vi "Arm Solenoid.vi"(10 "Value":T1, 11 "Enum":enum16{"Start", "Run", "End"}(ring)=enum."Run") -> ()   [LabVIEW 2012]
uses:
  TypeDefs/Solenoid Module 1.ctl
  <vilib>/Rock Robotics/WPI/Solenoid/WPI_SolenoidChannel.ctl
  <vilib>/Rock Robotics/SystemInterfaces/Typedef/FPGA_TypedefSolenoidModule.ctl
  <vilib>/Rock Robotics/WPI/Solenoid/WPI_SolenoidValue.ctl
  <vilib>/Rock Robotics/WPI/Solenoid/WPI_SolenoidOpenDouble.vi
  <vilib>/Rock Robotics/WPI/Solenoid/WPI_SolenoidSetEnum.vi
panel:
  in  "Solenoid Module 1":T2={"Lock Arm"=enum."Solenoid 1", "Shoot FWD"=enum."Solenoid 2", "Shoot REV"=enum."Solenoid 3", "Tip FWD"=enum."Solenoid 4", "Tip REV"=enum."Solenoid 5", "Unassigned"=enum."Solenoid 6", "Unassigned"=enum."Solenoid 7", "Unassigned"=enum."Solenoid 8", "Module"=enum."Solenoid Module 1"}
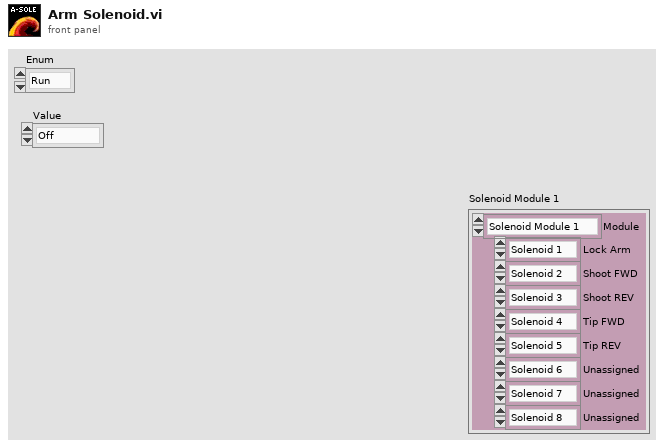
[diagram p1: front panel]
types:
  T1 = typedef "WPI_SolenoidValue.ctl" = enum16{"Off", "On", "Forward", "Reverse"}
  T2 = typedef "Solenoid Module 1.ctl" = cluster{"Lock Arm":T3, "Shoot FWD":T3, "Shoot REV":T3, "Tip FWD":T3, "Tip REV":T3, "Unassigned":T3, "Unassigned":T3, "Unassigned":T3, "Module":T4}
  T3 = typedef "WPI_SolenoidChannel.ctl" = enum8{"Solenoid 1", "Solenoid 2", "Solenoid 3", "Solenoid 4", "Solenoid 5", "Solenoid 6", "Solenoid 7", "Solenoid 8", "Invalid"}
  T4 = typedef "FPGA_TypedefSolenoidModule.ctl" = enum16{"Solenoid Module 1", "Solenoid Module 2"}
  T5 = typedef "WPI_SolenoidDevRef.ctl" = cluster{"DevStatus":errorcluster, "Solenoid Module":T4, "Forward Solenoid Channel":T3, "Reverse Solenoid Channel":T3}
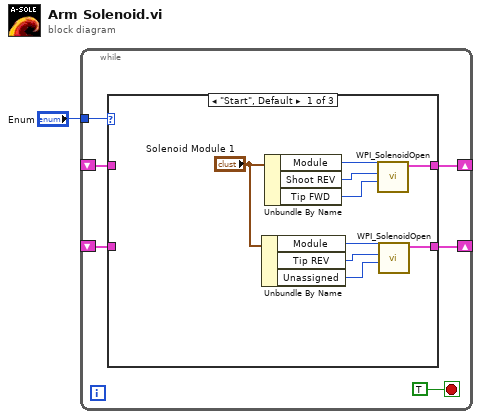
[diagram p0: block diagram]
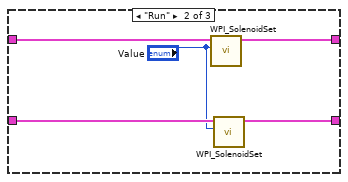
[diagram p2: hidden frame]
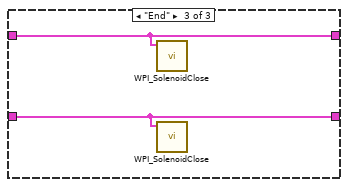
[diagram p3: hidden frame]
diagram:
  n1 = while {
    shift-right: [w7] -> _
    shift-left: _ -> [w5]
    tunnel: "Enum" -> [w6]
    shift-right: [w3] -> _
    shift-left: _ -> [w2]
    stop <- TRUE stop-if-true
    n2 = case shown="\"Start\", Default" w6 {
      tunnel: [w16 w21 w23] -> w7
      tunnel: w5 -> [_ w20 w23]
      tunnel: [w9 w19 w22] -> w3
      tunnel: w2 -> [_ w18 w22]
      frame "Start", Default {
        n3 = Unbundle By Name("Solenoid Module 1") -> ("Module"=w12:T4, "Tip REV"=w11:T3, "Unassigned"=w10:T3)
        n4 = Unbundle By Name("Solenoid Module 1") -> ("Module"=w15:T4, "Shoot REV"=w14:T3, "Tip FWD"=w13:T3)
        n5 = call-poly <vilib>:"WPI_SolenoidOpen.vi"("Reverse Solenoid Channel"=w13, "Forward Solenoid Channel"=w14, "Solenoid Module (Module 1)"=w15) -> ("SolenoidDevRef"=w16:T5)  [unwired: 7 in, 1 out]
        n6 = call-poly <vilib>:"WPI_SolenoidOpen.vi"("Reverse Solenoid Channel"=w10, "Forward Solenoid Channel"=w11, "Solenoid Module (Module 1)"=w12) -> ("SolenoidDevRef"=w9:T5)  [unwired: 7 in, 1 out]
      }
      frame "Run" {
        n7 = call-poly <vilib>:"WPI_SolenoidSet.vi"("Value"="Value", "SolenoidDevRef"=w20) -> ("SolenoidDevRef"=w21:T5)  [unwired: 8 in, 1 out]
        n8 = call-poly <vilib>:"WPI_SolenoidSet.vi"("Value"="Value", "SolenoidDevRef"=w18) -> ("SolenoidDevRef"=w19:T5)  [unwired: 8 in, 1 out]
      }
      frame "End" {
        n9 = call <vilib>:"WPI_SolenoidClose.vi"("SolenoidDevRef"=w23) -> ()  [unwired: 10 in, 1 out]
        n10 = call <vilib>:"WPI_SolenoidClose.vi"("SolenoidDevRef"=w22) -> ()  [unwired: 10 in, 1 out]
      }
    }
  }
